vi "MiniPNewXmlBuild.vi"(1 "KALIP SEÇİMİ":i32(listbox)=5, 8 "error in":errorcluster, 9 "XMLinput":string, 10 "Ürün İsmi":string="deneme6", 11 "Path":path=path "C:/Test_Program") -> (0 "error out":errorcluster, 2 "Kalıparr":string[](array[string]))   [LabVIEW 2021]
uses:
  <vilib>/Utility/xml.llb/Write to XML File(string).vi
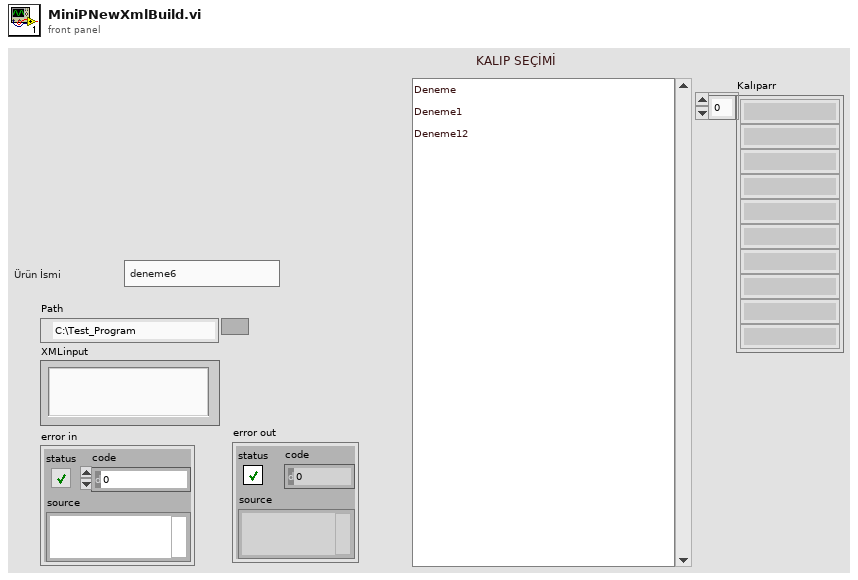
[diagram p1: front panel]
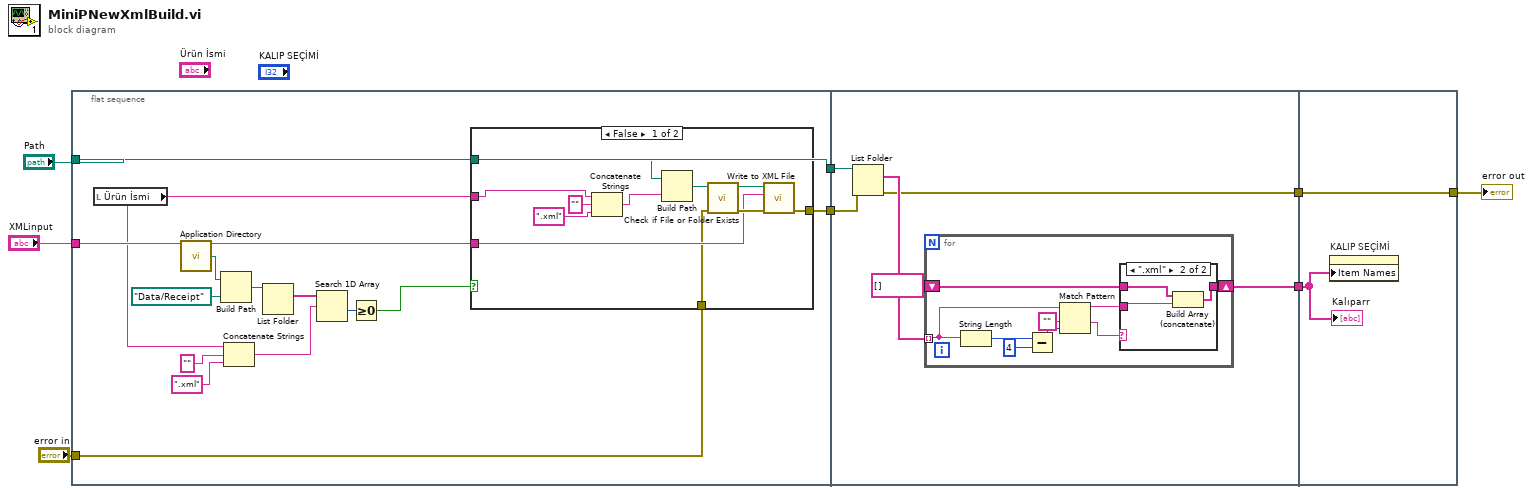
[diagram p0: block diagram]
diagram:
  n1 = flat-sequence {
    tunnel: "Path" -> [w19]
    tunnel: "XMLinput" -> [w22]
    tunnel: "error in" -> [w21]
    tunnel: [w20] -> w5
    tunnel: [w19] -> w1
    tunnel: w5 -> [w39]
    tunnel: [w37] -> w3
    tunnel: [w36] -> w2
    tunnel: w1 -> [w35]
    tunnel: [w55] -> w4
    tunnel: w3 -> [w55]
    tunnel: w2 -> [w54]
    frame #0 {
      n2 = local read "Ürün İsmi"() -> (w9:string)
      n3 = call <vilib>:"Application Directory.vi"() -> ("Application Directory"=w17:path)
      n4 = Build Path(base path=w17, name or relative path=path "Data/Receipt") -> (appended path=w13:path)
      n5 = Concatenate Strings(w9, "", ".xml") -> (w11:string)
      n6 = List Folder(path=w13) -> (filenames=w12:string[])  [unwired: 3 in, 3 out]
      n7 = Search 1D Array(1D array=w12, element=w11) -> (index of element=w14:i32)  [unwired: 1 in]
      n8 = Greater Or Equal To 0?(x=w14) -> (x >= 0?=w10:bool)
      n9 = case shown="False" w10 {
        tunnel: w22 -> [w30 _]
        tunnel: w21 -> [w29 w34]
        tunnel: [w28 w34] -> w20
        tunnel: w19 -> [w27 _]
        tunnel: w9 -> [w26 _]
        frame False {
          n10 = Concatenate Strings(w26, "" ("string"), ".xml" ("string")) -> (w23:string)
          n11 = Build Path(base path=w27, name or relative path=w23) -> (appended path=w33:path)
          n12 = call <vilib>:"Check if File or Folder Exists.vi"("error in (no error)"=w29, "path"=w33) -> ("error out"=w31:errorcluster, "dup path"=w32:path)  [unwired: 7 in, 1 out]
          n13 = call-poly <vilib>:"Write to XML File.vi"("error in (no error)"=w31, "XML Input"=w30, "XML File Path"=w32) -> ("error out"=w28:errorcluster)  [unwired: 6 in, 2 out]
        }
        frame True {
        }
      }
    }
    frame #1 {
      n14 = List Folder(path=w35, error in=w39) -> (filenames=w40:string[], error out=w37:errorcluster)  [unwired: 2 in, 2 out]
      n15 = for {
        tunnel: w40 -> [w41] mode=indexing
        shift-right: [w45] -> w36
        shift-left: string[] [] -> [w46]
        n16 = String Length(string=w41) -> (length=w44:i32)
        n17 = Subtract(x=w44, y=4) -> (x-y=w42:i32)
        n18 = Match Pattern(string=w41, regular expression="", offset (0)=w42) -> (before substring=w47:string, after substring=w48:string)  [unwired: 2 out]
        n19 = case shown="\".xml\"" w48 {
          tunnel: w47 -> [_ w51]
          tunnel: w46 -> [w50 w53]
          tunnel: [w50 w52] -> w45
          frame "False", Default {
          }
          frame ".xml" {
            n20 = Build Array (concatenate)(w53, w51) -> (w52:string[])
          }
        }
      }
    }
    frame #2 {
      n21 = property on="KALIP SEÇİMİ" class="LstBox (strict)"("Item Names"=w54) -> ()  [unwired: 2 in, 2 out]
      "Kalıparr" <- w54
    }
  }
  "error out" <- w4
